vi "time tokenize.vi"() -> ()   [LabVIEW 2014]
uses:
  layer.ctl
  processed node.ctl
  json node type.ctl
panel:
  out "layers":T1[](array[typedef])
  out "element":bool
  out "x-y":dbl=1.9602011889219284e-06
  in  "String":string="{\n    \"id\": 1,\n    \"name\": \"Foo\",\n    \"price\": 123,\n    \"tags\": [ \"Bar\", \"Eek\" ],\n    \"stock\": {\n        \"warehouse\": 300,\n        \"retail\": 20\n    }\n}"
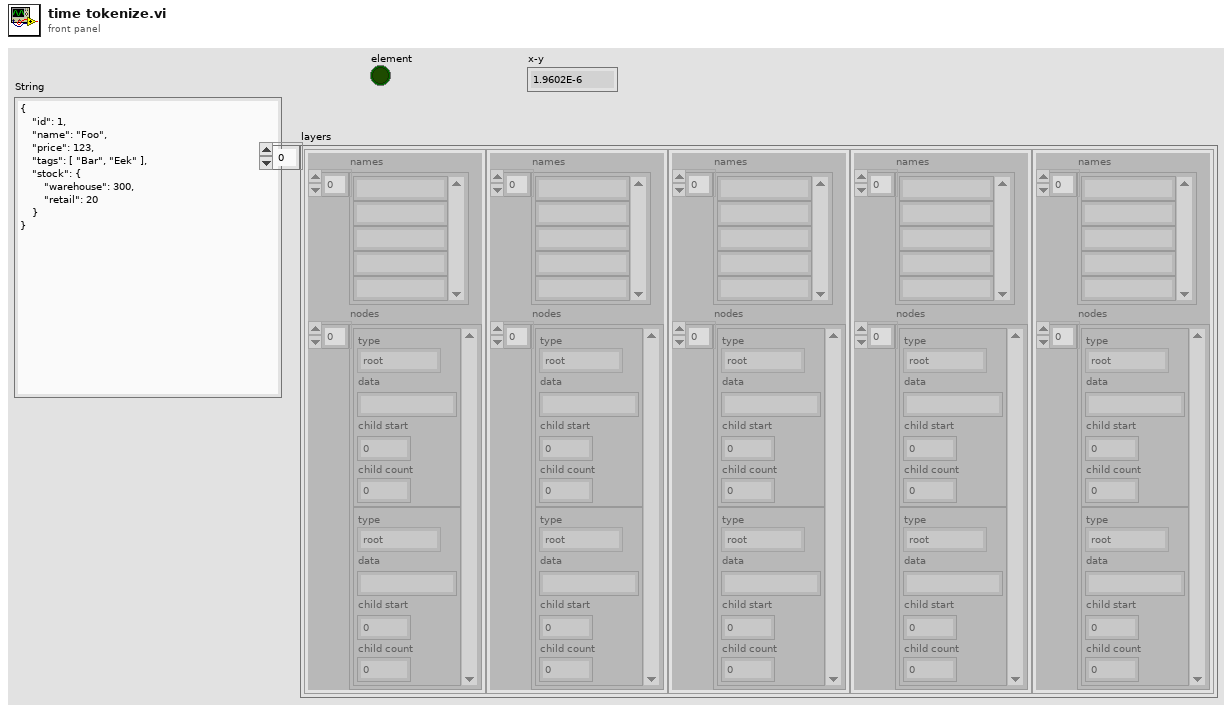
[diagram p1: front panel]
types:
  T1 = typedef "layer.ctl" = cluster{"names":string[], "nodes":T2[]}
  T2 = typedef "processed node.ctl" = cluster{"type":T3, "data":string, "child start":i32, "child count":i32}
  T3 = typedef "json node type.ctl" = enum16{"root", "object", "array", "number", "string value", "string key", "true", "false", "null"}
  T4 = typedef "json token.ctl" = cluster{"type":T3, "start":i32, "length":i32, "children (r, o, a)":u16, "parent (r=-1)":i32}
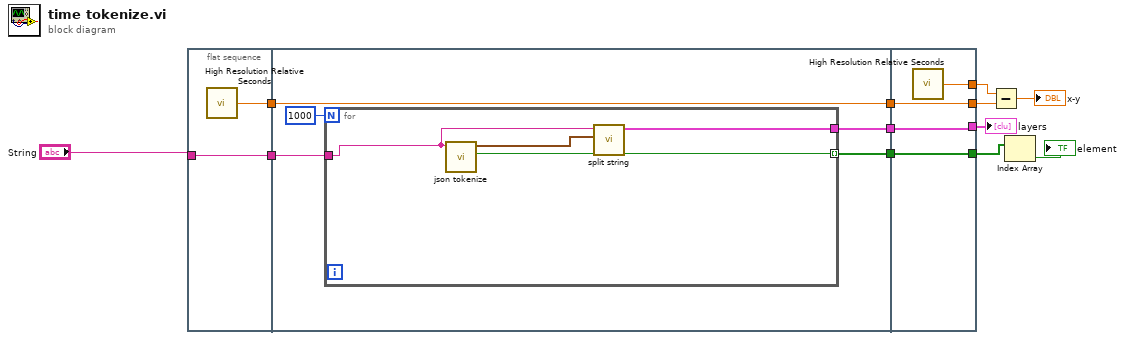
[diagram p0: block diagram]
diagram:
  n1 = flat-sequence {
    tunnel: "String" -> [w14]
    tunnel: [w14] -> w12
    tunnel: [w13] -> w10
    tunnel: w12 -> [w19]
    tunnel: w10 -> [w18]
    tunnel: [w18] -> w9
    tunnel: [w17] -> w4
    tunnel: [w15] -> w2
    tunnel: [w27] -> w11
    tunnel: w9 -> [w26]
    tunnel: [w26] -> w8
    tunnel: [w25] -> w5
    tunnel: w4 -> [w25]
    tunnel: [w24] -> w1
    tunnel: w2 -> [w24]
    frame #0 {
      n2 = call <vilib>:"High Resolution Relative Seconds.vi"() -> ("relative seconds"=w13:dbl)
    }
    frame #1 {
      n3 = for {
        N: 1000 ("Numeric") -> [_]
        tunnel: w19 -> [w21]
        tunnel: [w23] -> w17 mode=indexing
        tunnel: [w20] -> w15
        n4 = call "json tokenize.vi"("String"=w21) -> ("error"=w23:bool, "tokens"=w22:T4[])  [unwired: 9 in]
        n5 = call "split string.vi"("tokens"=w22, "String"=w21) -> ("layers"=w20:T1[])  [unwired: 9 in]
      }
    }
    frame #2 {
      n6 = call <vilib>:"High Resolution Relative Seconds.vi"() -> ("relative seconds"=w27:dbl)
    }
  }
  n7 = Subtract(x=w11, y=w8) -> (x-y=→"x-y":dbl)
  n8 = Index Array(array=w5) -> (element=→"element":bool)  [unwired: 1 in]
  "layers" <- w1
